vi "HP1200_061_set_IntSelLckd.vi"(7 "device_addr":u16=22, 8 "error in":errorcluster, 10 "onoff":enum16{"ON", "OFF"}(ring), 11 "conn_id_in":refnum<k5>) -> (0 "error out":errorcluster, 1 "response":string, 2 "onoff_ret":string, 3 "conn_id_out":refnum<k5>, 4 "status":bool)   [LabVIEW 2019]
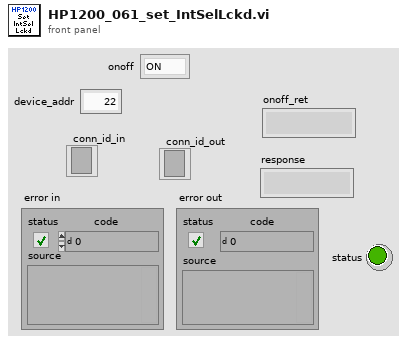
[diagram p1: front panel]
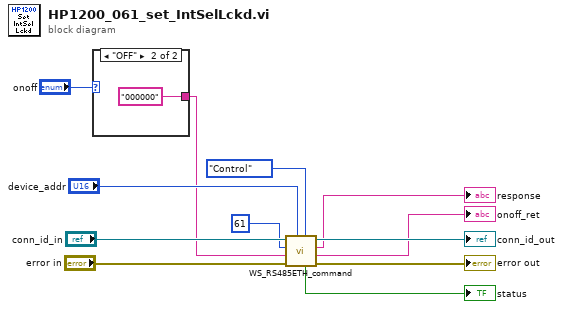
[diagram p0: block diagram]
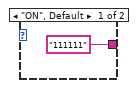
[diagram p2: hidden frame]
diagram:
  n1 = case shown="\"OFF\"" "onoff" {
    tunnel: ["111111" ("data") "000000" ("data")] -> w2
    frame "ON", Default {
    }
    frame "OFF" {
    }
  }
  n2 = call "WS_RS485ETH_command.vi"("action"=enum16{"Request", "Control"}."Control", "device_addr"="device_addr", "error in"="error in", "data_string"=w2, "param_num"=u16 61, "conn_id_in"="conn_id_in") -> ("error out"=→"error out":errorcluster, "data_out"=→"onoff_ret":string, "response"=→"response":string, "conn_id_out"=→"conn_id_out":refnum<k5>, "status"=→"status":bool)  [unwired: 1 in]
